vi "stabilizePress_03.vi"() -> ()   [LabVIEW 2011]
uses:
  <vilib>/Platform/TimedLoop/XDataNode/XDataNode.xnode
  <vilib>/Platform/TimedLoop/XDataNode/nitl_modes.ctl
  <vilib>/Platform/TimedLoop/XDataNode/XDNodeRunTimeDep.lvlib
  <vilib>/Platform/TimedLoop/XDataNode/wakeup.ctl
  <vilib>/Platform/TimedLoop/XDataNode/timing_clust.ctl
  <vilib>/Analysis/NI_AALPro.lvlib
panel:
  in  "dtRamp (s)":i64=2
  in  "local when done":bool=TRUE
  out "Best Exponential Fit":dbl[](array[numeric])=[20.391769446914367, 19.671893548435698, 19.339647975340863, 19.18630609922805, 19.115533956951577, 19.082870367269678, 19.067795084021366, 19.060832753073868, 19.057626153023538, 19.056144077997605, 19.055460053338074, 19.055144354249524, 19.05499864910115, 19.054931401551084, 19.054900364672562, 19.05488604016814, 19.054879428954745, 19.05487637564856, 19.054874969405184, 19.054874319446302, 19.05487401946965, 19.054873881020907]
  out "XY Graph":cluster{"Value":dbl[], "Value":dbl[]}[](graph)=[{"Value"=[1.0, 2.0, 3.0, 4.0, 5.0, 6.0, 7.0, 8.001, 9.0, 10.0, 11.0, 12.0, 13.0, 14.0, 15.0, 16.0, 17.0, 18.001, 19.0, 20.0, 21.0, 22.0], "Value"=[20.39, 19.689999999999998, 19.299999999999997, 19.189999999999998, 19.130000000000003, 19.110000000000003, 19.09, 19.08, 19.07, 19.05, 19.04, 19.04, 19.05, 19.05, 19.05, 19.04, 19.05, 19.060000000000002, 19.060000000000002, 19.05, 19.05, 19.05]}, {"Value"=[1.0, 2.0, 3.0, 4.0, 5.0, 6.0, 7.0, 8.001, 9.0, 10.0, 11.0, 12.0, 13.0, 14.0, 15.0, 16.0, 17.0, 18.001, 19.0, 20.0, 21.0, 22.0], "Value"=[20.391769446914367, 19.671893548435698, 19.339647975340863, 19.18630609922805, 19.115533956951577, 19.082870367269678, 19.067795084021366, 19.060832753073868, 19.057626153023538, 19.056144077997605, 19.055460053338074, 19.055144354249524, 19.05499864910115, 19.054931401551084, 19.054900364672562, 19.05488604016814, 19.054879428954745, 19.05487637564856, 19.054874969405184, 19.054874319446302, 19.05487401946965, 19.054873881020907]}]
  out "Pfinal (torr)":dbl=19.054873762353765
  out "tune done":bool=TRUE
  in  "max dP step (torr)":dbl=0.1
  out "dP(torr)":dbl
  out "amplitude":dbl=2.8966495268264136
  out "damping":dbl=-0.7732044604437537
  out "tune Setpoint(torr)":dbl=20.0
  in  "t array":dbl[](array[numeric])=[1.0, 2.0, 3.0, 4.0, 5.0, 6.0, 7.0, 8.001, 9.0, 10.0, 11.0, 12.0, 13.0, 14.0, 15.0, 16.0, 17.0, 18.001, 19.0, 20.0, 21.0, 22.0]
  out "P array":dbl[](array[numeric])=[20.39, 19.689999999999998, 19.299999999999997, 19.189999999999998, 19.130000000000003, 19.110000000000003, 19.09, 19.08, 19.07, 19.05, 19.04, 19.04, 19.05, 19.05, 19.05, 19.04, 19.05, 19.060000000000002, 19.060000000000002, 19.05, 19.05, 19.05]
  out "fit done":bool=TRUE
  in  "tFit(s)":dbl=20.0
  in  "dtFit (s)":i64=1
  out "Set Point (torr)":dbl=20.0 format="%.2f"
  out "Setpoint Index":string="C"
  out "Setpoint Index control":u16(ring)=2 caption="Setpoint" items=["A", "B", "C", "D"]
  out "first":bool
  out "tStart":dbl=22.0
  in  "time done (s)":dbl
  out "Wait to set":bool
  out "IO error":errorcluster
  in  "stop":bool
  out "P (torr)":dbl=19.05 format="%.2f"
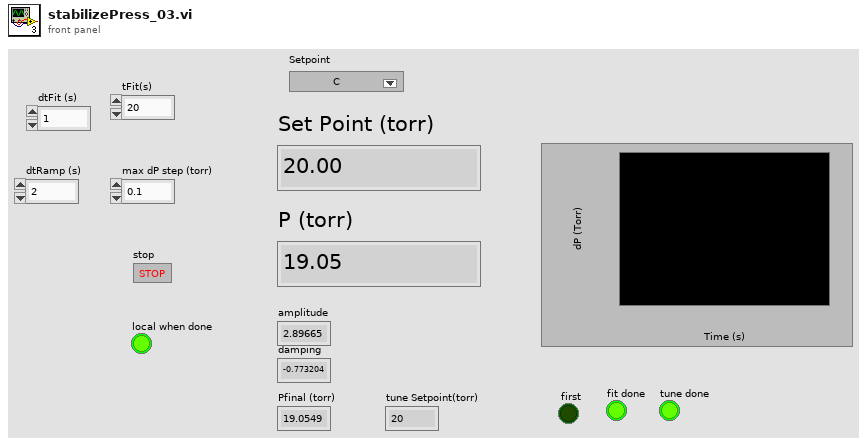
[diagram p1: front panel]
types:
  T1 = typedef "XDNodeRunTimeDep.lvlib/timing_clust.ctl" = cluster{"Expected End [f-1]":u64, "Actual End [f-1]":u64, "Finished Late? [f-1]":bool, "Expected End [i-1]":u64, "Actual End [i-1]":u64, "Finished Late? [i-1]":bool, "Expected Start [i]":u64, "Actual Start [i]":u64, "Expected Start [f]":u64, "Actual Start [f]":u64, "Source Name":string, "Structure Name":string, "Period":i64, "Deadline":i64, "Offset":i64, "Start":i64, "Priority":i32, "Timeout":i32, "Mode":T2, "Wakeup Reason":T3, "Error":errorcluster, "Source Type":string, "Secondary Source Type":string, "Global End Time":u64, "Global Start Time":u64, "Frame Duration":u64, "Iteration Duration":u64, "Assigned CPU":i32, "I/O Scan Engine Mode":u32}
  T2 = typedef "XDNodeRunTimeDep.lvlib/nitl_modes.ctl" = enum32{"No Change", "Process missed periods, maintain original phase", "Discard missed periods, maintain original phase", "Process missed periods, ignore original phase", "Discard missed periods, ignore original phase"}
  T3 = typedef "XDNodeRunTimeDep.lvlib/wakeup.ctl" = enum32{"Normal", "Aborted", "Asynchronous wakeup", "Timing source error", "Timed loop error", "Timeout"}
  T4 = cluster{"amp min":dbl, "amp max":dbl, "damping min":dbl, "damping max":dbl, "offset min":dbl, "offset max":dbl}
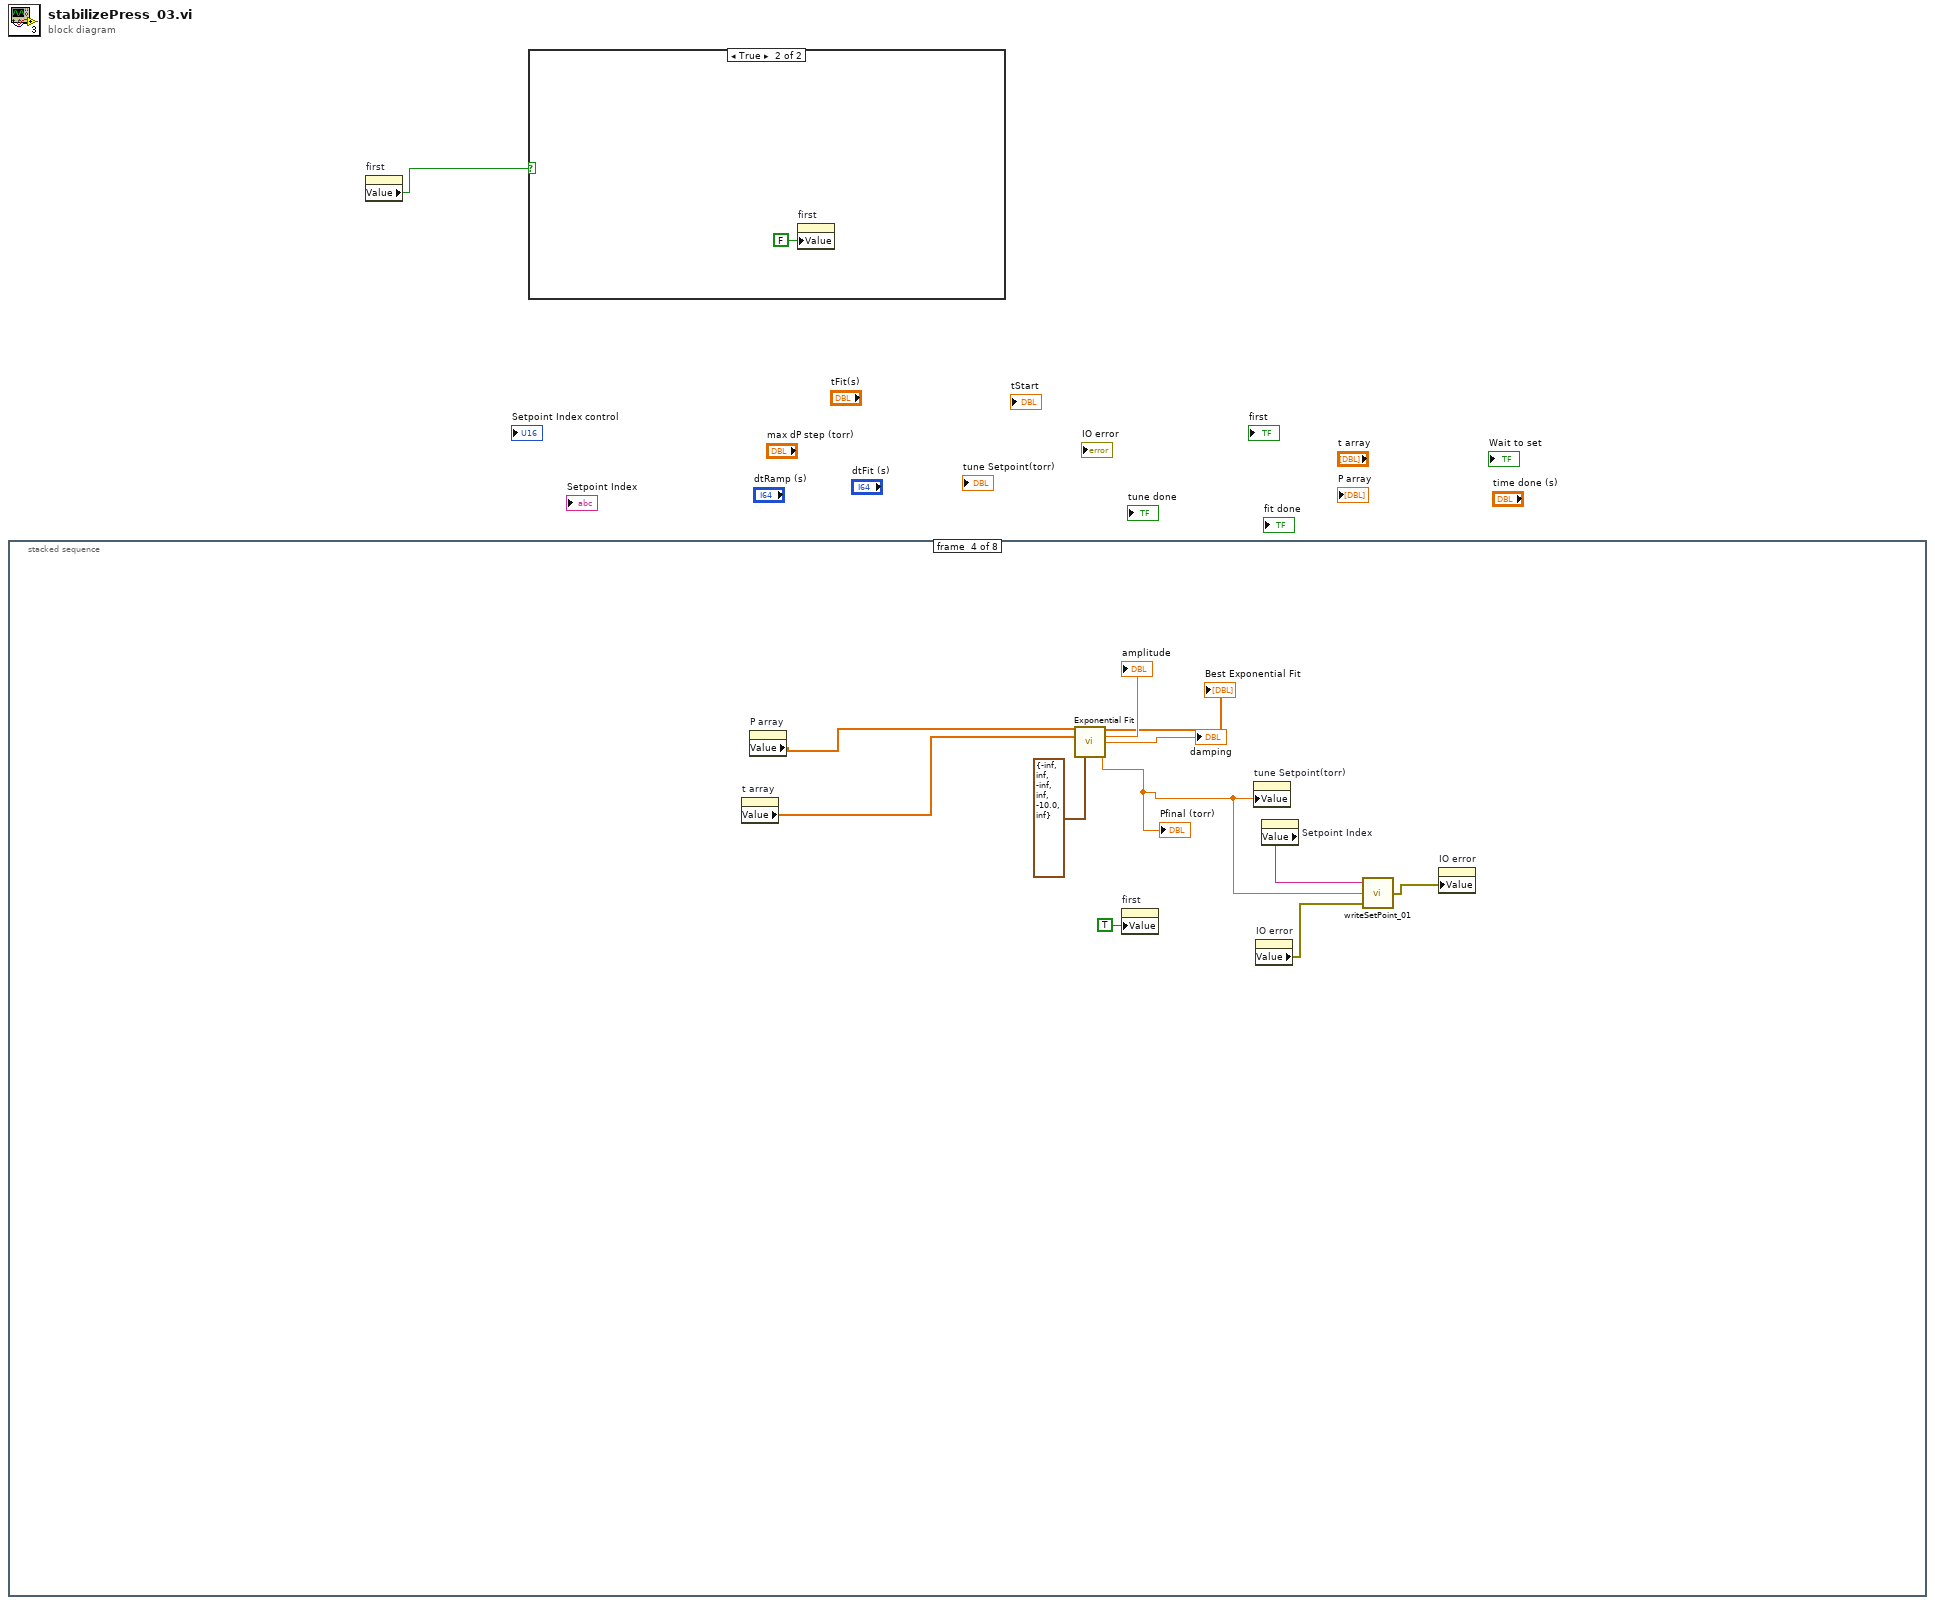
[diagram p0: block diagram]
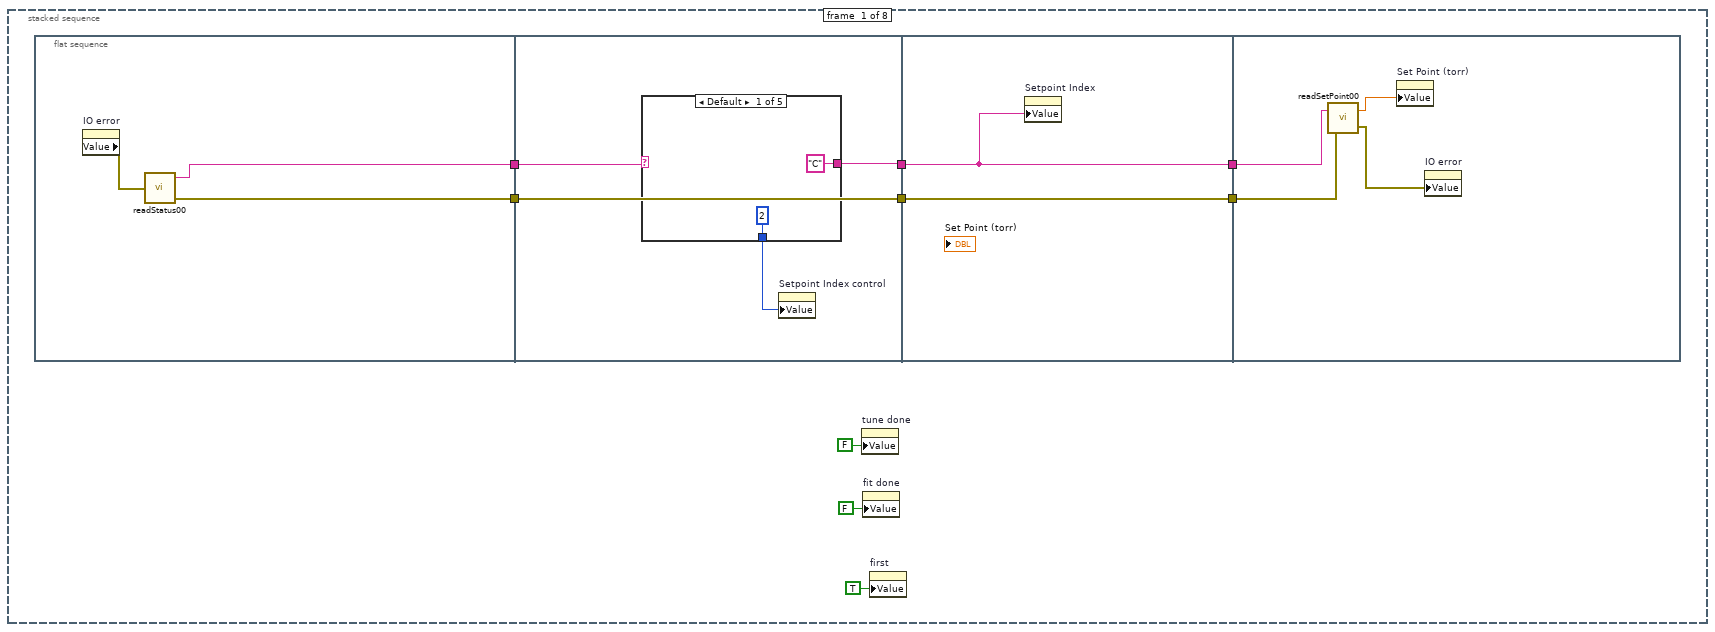
[diagram p3: hidden frame]
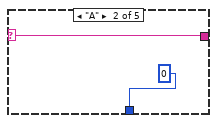
[diagram p4: hidden frame]
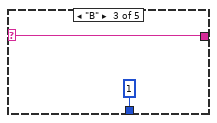
[diagram p5: hidden frame]
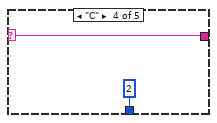
[diagram p6: hidden frame]
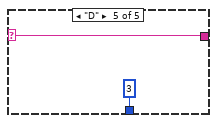
[diagram p7: hidden frame]
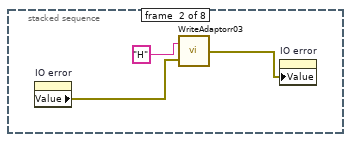
[diagram p8: hidden frame]
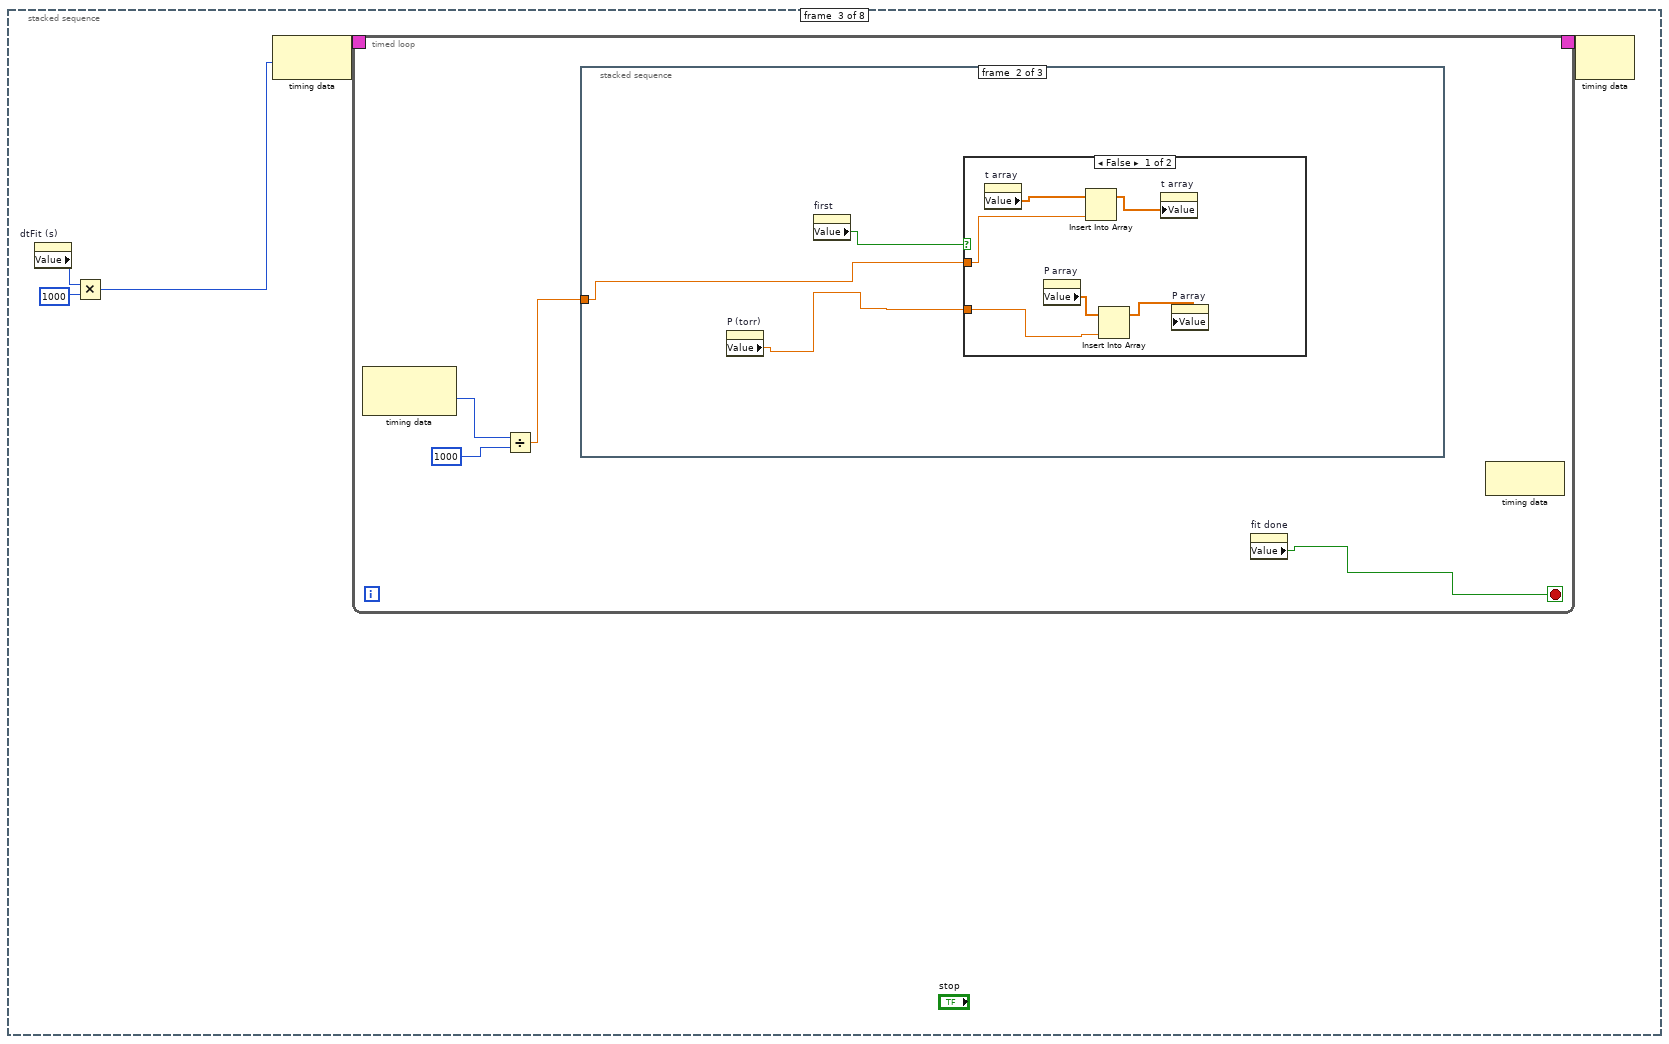
[diagram p9: hidden frame]
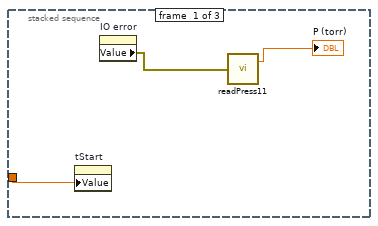
[diagram p10: hidden frame]
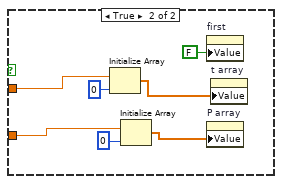
[diagram p11: hidden frame]
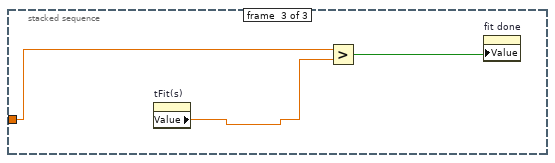
[diagram p12: hidden frame]
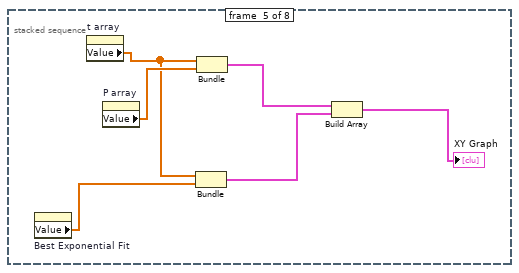
[diagram p13: hidden frame]
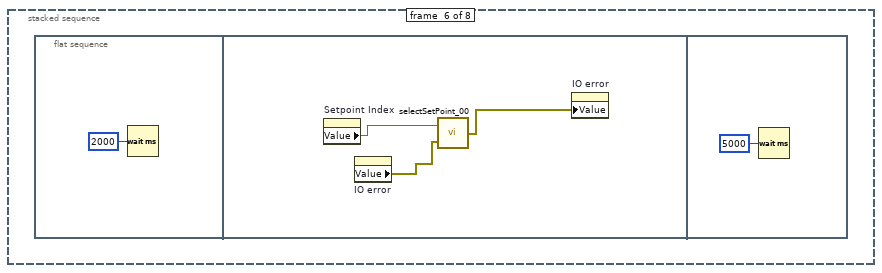
[diagram p14: hidden frame]
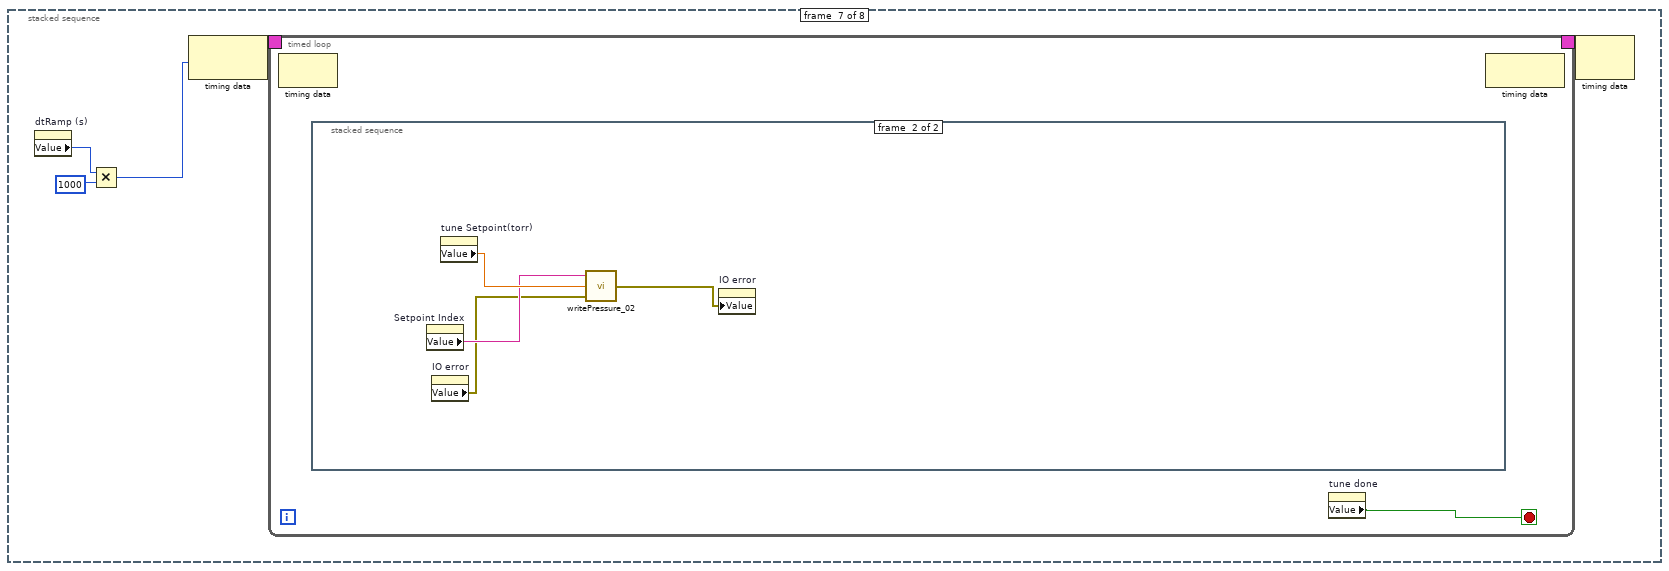
[diagram p15: hidden frame]
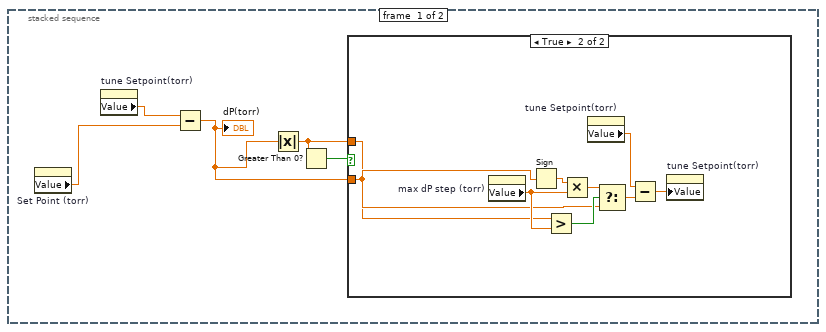
[diagram p16: hidden frame]
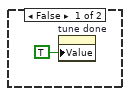
[diagram p17: hidden frame]
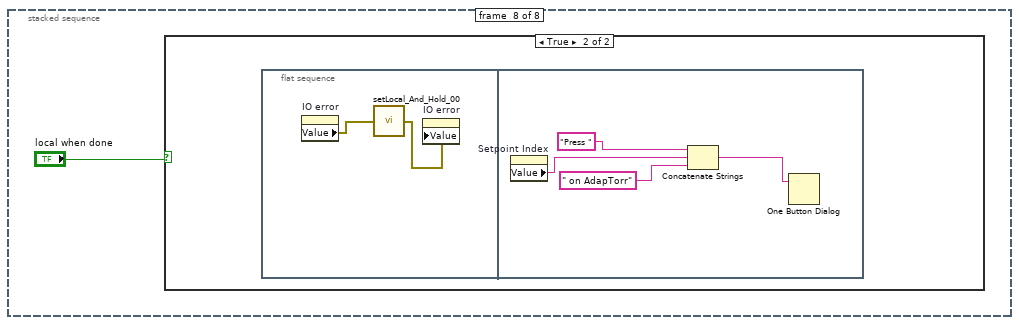
[diagram p18: hidden frame]
diagram:
  n1 = stacked-sequence {
    frame #0 {
      n2 = flat-sequence {
        tunnel: [w12] -> w10
        tunnel: [w11] -> w9
        tunnel: w10 -> [w16]
        tunnel: [w15] -> w8
        tunnel: w9 -> [w17]
        tunnel: [w17] -> w7
        tunnel: w8 -> [w28]
        tunnel: [w28] -> w6
        tunnel: w7 -> [w29]
        tunnel: [w29] -> w5
        tunnel: w6 -> [w33]
        tunnel: w5 -> [w32]
        frame #0 {
          n3 = property on="IO error" class="Clust (strict)"() -> ("Value"=w13:errorcluster)  [unwired: 2 in, 2 out]
          n4 = call "readStatus00.vi"("error in"=w13) -> ("Setpoint"=w12:string, "error out"=w11:errorcluster)  [unwired: 1 out]
        }
        frame #1 {
          n5 = case shown="Default" w16 {
            selector: w16 -> [_ w21 w22 w24 w26]
            tunnel: ["C" w21 w22 w24 w26] -> w15
            tunnel: [u16 2 ("Ring") u16 0 ("Ring") u16 1 ("Ring") u16 2 ("Ring") u16 3 ("Ring")] -> w14
            frame Default {
            }
            frame "A" {
            }
            frame "B" {
            }
            frame "C" {
            }
            frame "D" {
            }
          }
          n6 = property on="Setpoint Index control" class="Ring (strict)"("Value"=w14) -> ()  [unwired: 2 in, 2 out]
        }
        frame #2 {
          n7 = property on="Setpoint Index" class="Str"("Value"=w28) -> ()  [unwired: 2 in, 2 out]
        }
        frame #3 {
          n8 = call "readSetPoint00.vi"("error in"=w32, "Setpoint"=w33) -> ("error out"=w31:errorcluster, "P"=w30:dbl)
          n9 = property on="Set Point (torr)" class="DigNum (strict)"("Value"=w30) -> ()  [unwired: 2 in, 2 out]
          n10 = property on="IO error" class="Clust (strict)"("Value"=w31) -> ()  [unwired: 2 in, 2 out]
        }
      }
      n11 = property on="tune done" class="Bool (strict)"("Value"=FALSE ("tune done")) -> ()  [unwired: 2 in, 2 out]
      n12 = property on="fit done" class="Bool (strict)"("Value"=FALSE ("fit done")) -> ()  [unwired: 2 in, 2 out]
      n13 = property on="first" class="Bool (strict)"("Value"=TRUE ("first")) -> ()  [unwired: 2 in, 2 out]
    }
    frame #1 {
      n14 = property on="IO error" class="Clust (strict)"() -> ("Value"=w35:errorcluster)  [unwired: 2 in, 2 out]
      n15 = call "WriteAdaptorr03.vi"("error in (no error)"=w35, "string to write"="H") -> ("error out"=w34:errorcluster)
      n16 = property on="IO error" class="Clust (strict)"("Value"=w34) -> ()  [unwired: 2 in, 2 out]
    }
    frame #2 {
      n17 = property on="dtFit (s)" class="DigNum (strict)"() -> ("Value"=w38:i64)  [unwired: 2 in, 2 out]
      n18 = Multiply(x=w38, y=u32 1000) -> (x*y=w37:i64)
      n19 = node-c288(w37) -> (w41:T1)
      n20 = timed-loop {
        timing: w41 -> [_]
        timing-out: [_] -> w40
        stop <- w42 stop-if-true
        n21 = node-c288() -> (w45:i64)  [unwired: 1 in, 1 out]
        n22 = Divide(x=w45, y=i64 1000) -> (x/y=w43:dbl)
        n23 = stacked-sequence {
          tunnel: w43 -> [w48 w49 w67]
          frame #0 {
            n24 = property on="tStart" class="DigNum (strict)"("Value"=w48) -> ()  [unwired: 2 in, 2 out]
            n25 = property on="IO error" class="Clust (strict)"() -> ("Value"=w46:errorcluster)  [unwired: 2 in, 2 out]
            n26 = call "readPress11.vi"("error in"=w46) -> ("P"=→"P (torr)":dbl)  [unwired: 1 out]
          }
          frame #1 {
            n27 = property on="P (torr)" class="DigNum (strict)"() -> ("Value"=w50:dbl)  [unwired: 2 in, 2 out]
            n28 = property on="first" class="Bool (strict)"() -> ("Value"=w51:bool)  [unwired: 2 in, 2 out]
            n29 = case shown="False" w51 {
              tunnel: w50 -> [w57 w63]
              tunnel: w49 -> [w54 w61]
              frame False {
                n30 = property on="t array" class="Arr (strict)"() -> ("Value"=w53:dbl[])  [unwired: 2 in, 2 out]
                n31 = property on="P array" class="Arr (strict)"() -> ("Value"=w55:dbl[])  [unwired: 2 in, 2 out]
                n32 = Insert Into Array(array=w53, new element=w54) -> (w52:dbl[])  [unwired: 1 in]
                n33 = Insert Into Array(array=w55, new element=w57) -> (w56:dbl[])  [unwired: 1 in]
                n34 = property on="t array" class="Arr (strict)"("Value"=w52) -> ()  [unwired: 2 in, 2 out]
                n35 = property on="P array" class="Arr (strict)"("Value"=w56) -> ()  [unwired: 2 in, 2 out]
              }
              frame True {
                n36 = Initialize Array(w61, 0 ("dimension size")) -> (w58:dbl[])
                n37 = Initialize Array(w63, 0 ("dimension size")) -> (w59:dbl[])
                n38 = property on="first" class="Bool (strict)"("Value"=FALSE ("first")) -> ()  [unwired: 2 in, 2 out]
                n39 = property on="P array" class="Arr (strict)"("Value"=w59) -> ()  [unwired: 2 in, 2 out]
                n40 = property on="t array" class="Arr (strict)"("Value"=w58) -> ()  [unwired: 2 in, 2 out]
              }
            }
          }
          frame #2 {
            n41 = property on="tFit(s)" class="DigNum (strict)"() -> ("Value"=w65:dbl)  [unwired: 2 in, 2 out]
            n42 = Greater?(x=w67, y=w65) -> (0:w66:bool)
            n43 = property on="fit done" class="Bool (strict)"("Value"=w66) -> ()  [unwired: 2 in, 2 out]
          }
        }
        n44 = property on="fit done" class="Bool (strict)"() -> ("Value"=w42:bool)  [unwired: 2 in, 2 out]
        n45 = node-c288() -> ()  [unwired: 1 in, 1 out]
      }
      n46 = node-c288(w40) -> ()  [unwired: 1 out]
    }
    frame #3 {
      n47 = property on="t array" class="Arr (strict)"() -> ("Value"=w84:dbl[])  [unwired: 2 in, 2 out]
      n48 = property on="P array" class="Arr (strict)"() -> ("Value"=w85:dbl[])  [unwired: 2 in, 2 out]
      n49 = call <vilib>:"Exponential Fit.vi"("Y"=w85, "X"=w84, "parameter bounds"=T4 {"amp min"=-inf, "amp max"=inf, "damping min"=-inf, "damping max"=inf, "offset min"=-10.0, "offset max"=inf}) -> ("Best Exponential Fit"=→"Best Exponential Fit":dbl[], "amplitude"=→"amplitude":dbl, "damping"=→"damping":dbl, "offset"=w78:dbl)  [unwired: 7 in, 2 out]
      "Pfinal (torr)" <- w78
      n50 = property on="first" class="Bool (strict)"("Value"=TRUE ("first")) -> ()  [unwired: 2 in, 2 out]
      n51 = property on="tune Setpoint(torr)" class="DigNum (strict)"("Value"=w78) -> ()  [unwired: 2 in, 2 out]
      n52 = property on="IO error" class="Clust (strict)"() -> ("Value"=w76:errorcluster)  [unwired: 2 in, 2 out]
      n53 = property on="Setpoint Index" class="Str"() -> ("Value"=w77:string)  [unwired: 2 in, 2 out]
      n54 = call "writeSetPoint_01.vi"("error in"=w76, "P (Torr)"=w78, "Setpoint"=w77) -> ("error out"=w75:errorcluster)
      n55 = property on="IO error" class="Clust (strict)"("Value"=w75) -> ()  [unwired: 2 in, 2 out]
    }
    frame #4 {
      n56 = property on="Best Exponential Fit" class="Arr (strict)"() -> ("Value"=w89:dbl[])  [unwired: 2 in, 2 out]
      n57 = property on="t array" class="Arr (strict)"() -> ("Value"=w90:dbl[])  [unwired: 2 in, 2 out]
      n58 = property on="P array" class="Arr (strict)"() -> ("Value"=w91:dbl[])  [unwired: 2 in, 2 out]
      n59 = Bundle "Bundle"("Value"=w90, "Value"=w89) -> (w87:cluster{"Value":dbl[], "Value":dbl[]})  [unwired: 1 in]
      n60 = Bundle "Bundle"("Value"=w90, "Value"=w91) -> (w88:cluster{"Value":dbl[], "Value":dbl[]})  [unwired: 1 in]
      n61 = Build Array "Build Array"(w88, w87) -> (→"XY Graph":cluster{"Value":dbl[], "Value":dbl[]}[])
    }
    frame #5 {
      n62 = flat-sequence {
        frame #0 {
          n63 = Wait (ms)(milliseconds to wait=u32 2000) -> ()  [unwired: 1 out]
        }
        frame #1 {
          n64 = property on="Setpoint Index" class="Str"() -> ("Value"=w95:string)  [unwired: 2 in, 2 out]
          n65 = property on="IO error" class="Clust (strict)"() -> ("Value"=w94:errorcluster)  [unwired: 2 in, 2 out]
          n66 = call "selectSetPoint_00.vi"("error in"=w94, "Setpoint"=w95) -> ("error out"=w93:errorcluster)
          n67 = property on="IO error" class="Clust (strict)"("Value"=w93) -> ()  [unwired: 2 in, 2 out]
        }
        frame #2 {
          n68 = Wait (ms)(milliseconds to wait=u32 5000) -> ()  [unwired: 1 out]
        }
      }
    }
    frame #6 {
      n69 = property on="dtRamp (s)" class="DigNum (strict)"() -> ("Value"=w97:i64)  [unwired: 2 in, 2 out]
      n70 = Multiply(x=w97, y=u32 1000) -> (x*y=w98:i64)
      n71 = node-c288(w98) -> (w101:T1)
      n72 = timed-loop {
        timing: w101 -> [_]
        timing-out: [_] -> w100
        stop <- w102 stop-if-true
        n73 = node-c288() -> ()  [unwired: 1 in, 1 out]
        n74 = stacked-sequence {
          frame #0 {
            n75 = property on="Set Point (torr)" class="DigNum (strict)"() -> ("Value"=w107:dbl)  [unwired: 2 in, 2 out]
            n76 = property on="tune Setpoint(torr)" class="DigNum (strict)"() -> ("Value"=w106:dbl)  [unwired: 2 in, 2 out]
            n77 = Subtract(x=w106, y=w107) -> (x-y=w105:dbl)
            "dP(torr)" <- w105
            n78 = Absolute Value(x=w105) -> (abs(x)=w104:dbl)
            n79 = Greater Than 0?(x=w104) -> (x > 0?=w103:bool)
            n80 = case shown="True" w103 {
              tunnel: w105 -> [_ w113]
              tunnel: w104 -> [_ w109]
              frame False {
                n81 = property on="tune done" class="Bool (strict)"("Value"=TRUE ("tune done")) -> ()  [unwired: 2 in, 2 out]
              }
              frame True {
                n82 = property on="max dP step (torr)" class="DigNum (strict)"() -> ("Value"=w115:dbl)  [unwired: 2 in, 2 out]
                n83 = Sign(1:w113) -> (0:w116:dbl)
                n84 = Greater?(x=w109, y=w115) -> (0:w117:bool)
                n85 = Multiply(x=w116, y=w115) -> (x*y=w114:dbl)
                n86 = property on="tune Setpoint(torr)" class="DigNum (strict)"() -> ("Value"=w112:dbl)  [unwired: 2 in, 2 out]
                n87 = Select(t=w114, s=w117, f=w113) -> (s? t:f=w111:dbl)
                n88 = Subtract(x=w112, y=w111) -> (x-y=w110:dbl)
                n89 = property on="tune Setpoint(torr)" class="DigNum (strict)"("Value"=w110) -> ()  [unwired: 2 in, 2 out]
              }
            }
          }
          frame #1 {
            n90 = property on="Setpoint Index" class="Str"() -> ("Value"=w120:string)  [unwired: 2 in, 2 out]
            n91 = property on="IO error" class="Clust (strict)"() -> ("Value"=w119:errorcluster)  [unwired: 2 in, 2 out]
            n92 = property on="tune Setpoint(torr)" class="DigNum (strict)"() -> ("Value"=w121:dbl)  [unwired: 2 in, 2 out]
            n93 = call "writePressure_02.vi"("error in"=w119, "P (Torr)"=w121, 3:w120) -> ("error out"=w118:errorcluster)
            n94 = property on="IO error" class="Clust (strict)"("Value"=w118) -> ()  [unwired: 2 in, 2 out]
          }
        }
        n95 = property on="tune done" class="Bool (strict)"() -> ("Value"=w102:bool)  [unwired: 2 in, 2 out]
        n96 = node-c288() -> ()  [unwired: 1 in, 1 out]
      }
      n97 = node-c288(w100) -> ()  [unwired: 1 out]
    }
    frame #7 {
      n98 = case shown="True" "local when done" {
        frame False {
        }
        frame True {
          n99 = flat-sequence {
            frame #0 {
              n100 = property on="IO error" class="Clust (strict)"() -> ("Value"=w130:errorcluster)  [unwired: 2 in, 2 out]
              n101 = call "setLocal_And_Hold_00.vi"("error in (no error)"=w130) -> ("error out"=w129:errorcluster)
              n102 = property on="IO error" class="Clust (strict)"("Value"=w129) -> ()  [unwired: 2 in, 2 out]
            }
            frame #1 {
              n103 = property on="Setpoint Index" class="Str"() -> ("Value"=w132:string)  [unwired: 2 in, 2 out]
              n104 = Concatenate Strings("Press ", w132, " on AdapTorr") -> (w131:string)
              n105 = One Button Dialog(message=w131) -> ()  [unwired: 1 in, 1 out]
            }
          }
        }
      }
    }
  }
  n106 = property on="first" class="Bool (strict)"() -> ("Value"=w1:bool)  [unwired: 2 in, 2 out]
  n107 = case shown="True" w1 {
    frame False {
    }
    frame True {
      n108 = property on="first" class="Bool (strict)"("Value"=FALSE ("first")) -> ()  [unwired: 2 in, 2 out]
    }
  }
